vi "ConfigureDigitizer.vi"(7 "Software Trig?":bool, 8 "error in (no error)":errorcluster, 9 "# Samples after Trig":u16, 10 "handle":i32, 11 "VME Base Address":u32) -> (0 "error out":errorcluster, 3 "handle out":i32, 5 "VME Base Address out":u32)   [LabVIEW 2014]
uses:
  Program Files (x86)/CAEN/Comm/labview/CAENComm.lvlib
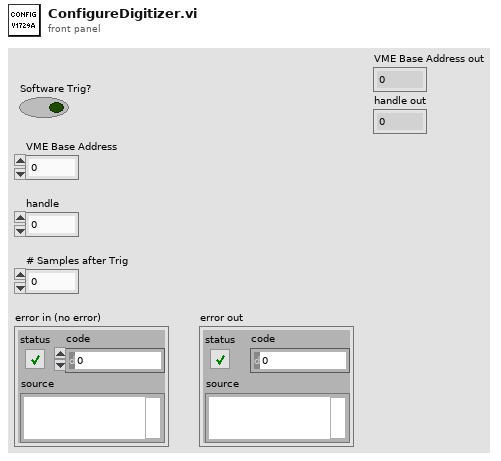
[diagram p1: front panel]
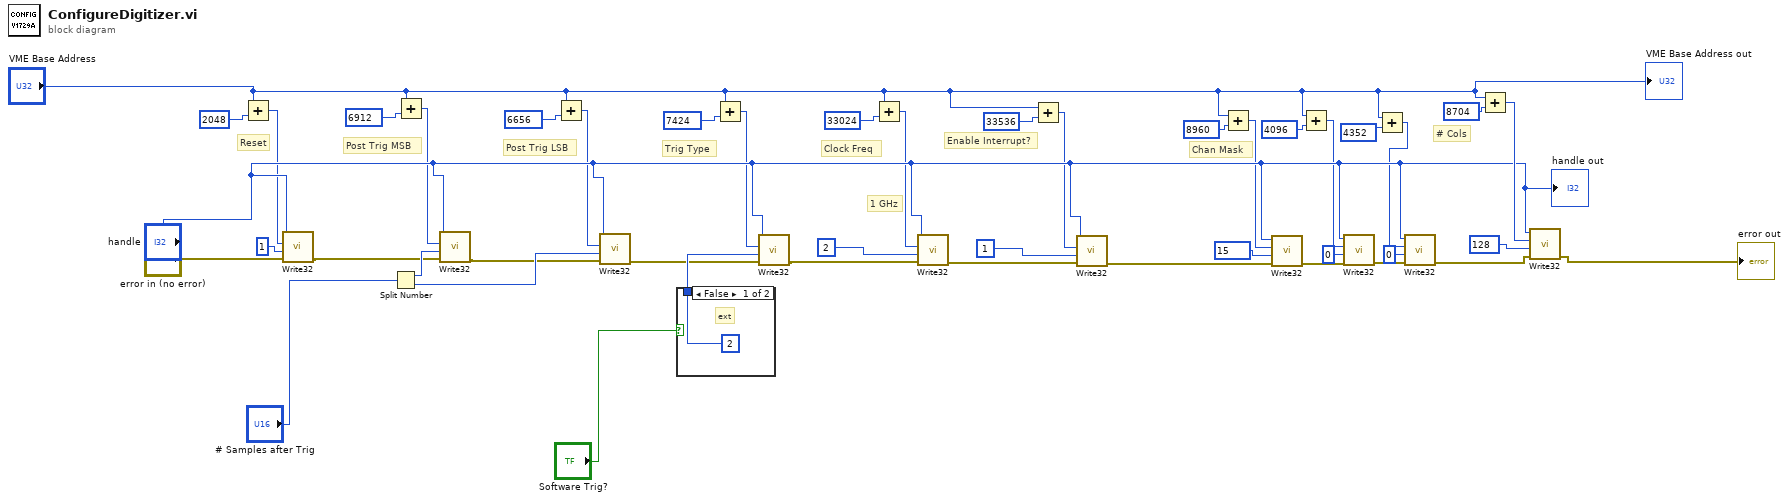
[diagram p0: block diagram]
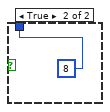
[diagram p2: hidden frame]
diagram:
  # "# Cols"
  # "Chan Mask"
  # "Enable Interrupt?"
  # "1 GHz"
  # "Clock Freq"
  # "Trig Type"
  # "Post Trig LSB"
  # "Post Trig MSB"
  # "Reset"
  n1 = Add(x="VME Base Address", y=u32 2048 ("x")) -> (x+y=w2:u32)
  n2 = call "Write32.vi"("error in (no error)"="error in (no error)", "Data"=u32 1, "Address"=w2, "handle"="handle") -> ("error out"=w7:errorcluster)  [unwired: 7 in]
  n3 = Split Number(x="# Samples after Trig") -> (hi(x)=w11:u8, lo(x)=w12:u8)
  n4 = Add(x="VME Base Address", y=u32 6912 ("x")) -> (x+y=w5:u32)
  n5 = call "Write32.vi"("error in (no error)"=w7, "Data"=w11, "Address"=w5, "handle"="handle") -> ("error out"=w10:errorcluster)  [unwired: 7 in]
  n6 = Add(x="VME Base Address", y=u32 6656 ("x")) -> (x+y=w8:u32)
  n7 = call "Write32.vi"("error in (no error)"=w10, "Data"=w12, "Address"=w8, "handle"="handle") -> ("error out"=w15:errorcluster)  [unwired: 7 in]
  n8 = case shown="False" "Software Trig?" {
    tunnel: [u8 2 ("Data") u8 8 ("Data")] -> w16
    frame False {
      # "ext"
    }
    frame True {
    }
  }
  n9 = Add(x="VME Base Address", y=u32 7424 ("x")) -> (x+y=w13:u32)
  n10 = call "Write32.vi"("error in (no error)"=w15, "Data"=w16, "Address"=w13, "handle"="handle") -> ("error out"=w20:errorcluster)  [unwired: 7 in]
  n11 = Add(x="VME Base Address", y=u32 33024 ("x")) -> (x+y=w17:u32)
  n12 = call "Write32.vi"("error in (no error)"=w20, "Data"=u8 2, "Address"=w17, "handle"="handle") -> ("error out"=w24:errorcluster)  [unwired: 7 in]
  n13 = Add(x="VME Base Address", y=u32 33536 ("x")) -> (x+y=w21:u32)
  n14 = call "Write32.vi"("error in (no error)"=w24, "Data"=u8 1, "Address"=w21, "handle"="handle") -> ("error out"=w37:errorcluster)  [unwired: 7 in]
  n15 = Add(x="VME Base Address", y=u32 8960 ("x")) -> (x+y=w26:u32)
  n16 = call "Write32.vi"("error in (no error)"=w37, "Data"=u8 15, "Address"=w26, "handle"="handle") -> ("error out"=w29:errorcluster)  [unwired: 7 in]
  n17 = Add(x="VME Base Address", y=u32 4096 ("x")) -> (x+y=w31:u32)
  n18 = call "Write32.vi"("error in (no error)"=w29, "Data"=u32 0, "Address"=w31, "handle"="handle") -> ("error out"=w33:errorcluster)  [unwired: 7 in]
  n19 = Add(x="VME Base Address", y=u32 4352 ("x")) -> (x+y=w35:u32)
  n20 = call "Write32.vi"("error in (no error)"=w33, "Data"=u32 0, "Address"=w35, "handle"="handle") -> ("error out"=w41:errorcluster)  [unwired: 7 in]
  n21 = Add(x="VME Base Address", y=u32 8704 ("x")) -> (x+y=w40:u32)
  n22 = call "Write32.vi"("error in (no error)"=w41, "Data"=u8 128, "Address"=w40, "handle"="handle") -> ("error out"=→"error out":errorcluster)  [unwired: 7 in]
  "VME Base Address out" <- "VME Base Address"
  "handle out" <- "handle"
